vi "SubVI_MixIntakeLiftTriggers_Teleop.vi"(11 "IntakeUp":bool) -> (1 "Lift+Lower":dbl)   [LabVIEW 2017]
uses:
  <vilib>/Rock Robotics/WPI/ThirdParty/Phoenix-LabVIEW/Motor Controller/Controls/CTRE_Phoenix_MotorControl_ControlMode.ctl
  <vilib>/Rock Robotics/WPI/ThirdParty/Phoenix-LabVIEW/Motor Controller/Get/CTRE_Phoenix_MotorController_GetSelectedSensorData.vi
panel:
  in  "Boolean":bool
  out "In Range?":bool
  in  "upper limit":dbl
  in  "lower limit":dbl=-5666.0
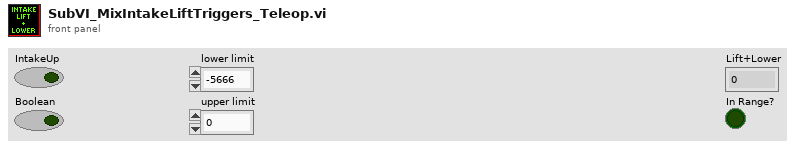
[diagram p1: front panel]
types:
  T1 = typedef "WPI_MotorControlDeviceRef.ctl" = cluster{"DeviceStatus":errorcluster, "Type":T2, "PWM":cluster{"PWM Channel":T3, "DeadBand":T4}, "CAN":cluster{"Device Number":u8, "SetOutput VI Ref":variant, "GetOutput VI Ref":variant, "Enable VI Ref":variant, "Disable VI Ref":variant, "Data":variant}, "Invert":bool, "DIO PWM":cluster{"PWM \"Enable\" Channel":T3, "DIOChannel":T5, "PWM Rate":dbl}}
  T2 = typedef "WPI_MotorControlType.ctl" = enum16{"PWM", "CAN", "DIO PWM"}
  T3 = typedef "FPGA_DIOPWMChannel.ctl" = enum8{"PWM 0", "PWM 1", "PWM 2", "PWM 3", "PWM 4", "PWM 5", "PWM 6", "PWM 7", "PWM 8", "PWM 9", "PWM MXP 0", "PWM MXP 1", "PWM MXP 2", "PWM MXP 3", "PWM MXP 4", "PWM MXP 5", "PWM MXP 6", "PWM MXP 7", "PWM MXP 8", "PWM MXP 9", "Invalid"}
  T4 = typedef "WPI_PWMDeadband.ctl" = cluster{"Name":string, "maxPositivePwm":i32, "minPositivePwm":i32, "centerPwm":i32, "maxNegativePwm":i32, "minNegativePwm":i32, "angularRange":u16}
  T5 = typedef "FPGA_DIOChannel.ctl" = enum8{"DIO 0", "DIO 1", "DIO 2", "DIO 3", "DIO 4", "DIO 5", "DIO 6", "DIO 7", "DIO 8", "DIO 9", "DIO MXP 0", "DIO MXP 1", "DIO MXP 2", "DIO MXP 3", "DIO MXP 4", "DIO MXP 5", "DIO MXP 6", "DIO MXP 7", "DIO MXP 8", "DIO MXP 9", "DIO MXP 10", "DIO MXP 11", "DIO MXP 12", "DIO MXP 13", "DIO MXP 14", "DIO MXP 15", "SPI Port CS1", "SPI Port CS2", "SPI Port CS3", "SPI Port MISO", "SPI Port MOSI", "Invalid"}
  T6 = typedef "CTRE_Phoenix_MotorControl_ControlMode.ctl" = u16
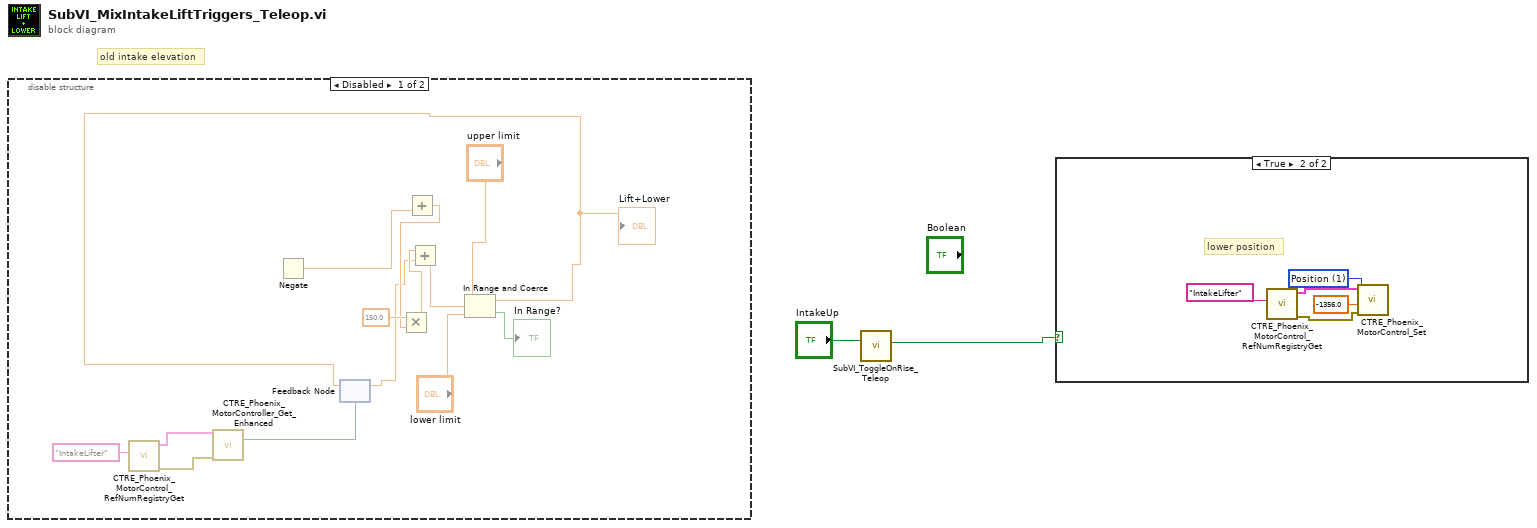
[diagram p0: block diagram]
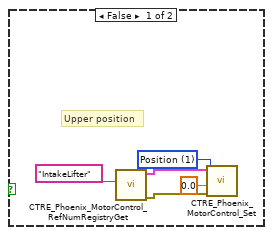
[diagram p2: hidden frame]
diagram:
  # "old intake elevation"
  n1 = disable-structure shown="Disabled" {
    frame Disabled {
      n2 = call <vilib>:"CTRE_Phoenix_MotorControl_RefNumRegistryGet.vi"("refnum name"="IntakeLifter") -> ("error out"=w14:errorcluster, "PhoenixMotorControlDevRef"=w15:T1)  [unwired: 9 in]
      n3 = call-poly <vilib>:"CTRE_Phoenix_MotorController_Get_Enhanced.vi"("PhoenixMotorControlDevRef"=w15, "error in"=w14) -> ("Position (Raw Sensor Units)"=w12:i32)  [unwired: 10 in, 3 out]
      n4 = Negate() -> (-x=w16:dbl)  [unwired: 1 in]
      n5 = feedback #1(w12) -> (w3:dbl)
      n6 = Add(y=w16) -> (x+y=w5:dbl)  [unwired: 1 in]
      n7 = Multiply(x=150.0, y=w5) -> (x*y=w4:dbl)
      n8 = Add(x=w4, y=w3) -> (x+y=w7:dbl)
      n9 = In Range and Coerce(upper limit="upper limit", x=w7, lower limit="lower limit") -> (coerced(x)=w8:dbl, In Range?=→"In Range?":bool)
      "Lift+Lower" <- w8
      n10 = feedback-in #1(w8) -> ()
    }
    frame Enabled {
    }
  }
  n11 = call "SubVI_ToggleOnRise_Teleop.vi"("Input"="IntakeUp") -> ("toggled"=w1:bool)  [unwired: 10 in]
  n12 = case shown="True" w1 {
    frame False {
      w17 = T6 1 items=["PercentOutput"=0, "Position"=1, "Velocity"=2, "Current"=3, "Follower"=5, "MotionProfile"=6, "MotionMagic"=7, "MotionMagicArc"=8, "MotionProfileArc"=10, "Disabled"=15] ("Control Mode")
      # "Upper position"
      n13 = call <vilib>:"CTRE_Phoenix_MotorControl_RefNumRegistryGet.vi"("refnum name"="IntakeLifter") -> ("error out"=w20:errorcluster, "PhoenixMotorControlDevRef"=w21:T1)  [unwired: 9 in]
      n14 = call <vilib>:"CTRE_Phoenix_MotorControl_Set.vi"("error in (no error)"=w20, "Output"=0.0, "Control Mode"=w17, "PhoenixMotorControlDevRef"=w21) -> ()  [unwired: 6 in, 2 out]
    }
    frame True {
      w24 = T6 1 items=["PercentOutput"=0, "Position"=1, "Velocity"=2, "Current"=3, "Follower"=5, "MotionProfile"=6, "MotionMagic"=7, "MotionMagicArc"=8, "MotionProfileArc"=10, "Disabled"=15] ("Control Mode")
      # "lower position"
      n15 = call <vilib>:"CTRE_Phoenix_MotorControl_RefNumRegistryGet.vi"("refnum name"="IntakeLifter") -> ("error out"=w22:errorcluster, "PhoenixMotorControlDevRef"=w26:T1)  [unwired: 9 in]
      n16 = call <vilib>:"CTRE_Phoenix_MotorControl_Set.vi"("error in (no error)"=w22, "Output"=-1356.0, "Control Mode"=w24, "PhoenixMotorControlDevRef"=w26) -> ()  [unwired: 6 in, 2 out]
    }
  }
